vi "Set VISA DBL output.vi"(7 "VISA resource name":refnum<visa-resource-name>, 8 "error in (no error)":errorcluster, 9 "Output value":dbl, 10 "Mag Lab Parameters in":refnum<class "Mag Lab Parameters.lvclass">, 11 "Keithley Current Source in":refnum<class "Keithley Current Source.lvclass">) -> (0 "error out":errorcluster, 1 "Actula output value":dbl, 3 "Keithley Current Source out":refnum<class "Keithley Current Source.lvclass">, 5 "VISA resource name out":refnum<visa-resource-name>)   [LabVIEW 2015, in "Keithley Current Source.lvclass"]
uses:
  Keithley Current Source.lvclass
  Mag Lab Properties/Mag Lab Parameters.lvclass
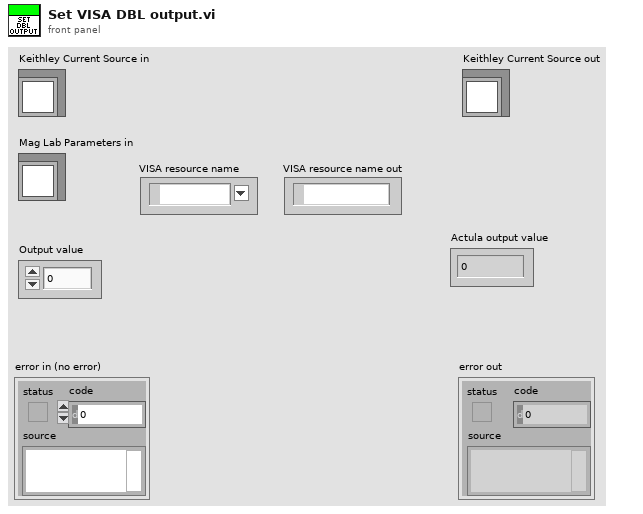
[diagram p1: front panel]
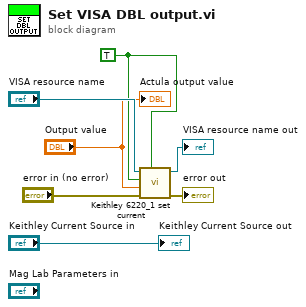
[diagram p0: block diagram]
diagram:
  w2 = TRUE ("Change output")
  n1 = call "Keithley 6220_1 set current.vi"("Change output"=w2, "error in (no error)"="error in (no error)", "Current (A)"="Output value", "Output ON"=w2, "VISA resource name"="VISA resource name") -> ("error out"=→"error out":errorcluster, "VISA resource name out"=→"VISA resource name out":refnum<visa-resource-name>)  [unwired: 5 in]
  "Keithley Current Source out" <- "Keithley Current Source in"
  "Actula output value" <- "Output value"
